vi "Mode_select_global_BM.vi"() -> ()   [LabVIEW 2021]
panel:
  in  "Mode Selection":T1(ring)
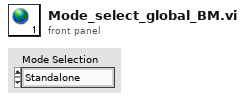
[diagram p1: front panel]
types:
  T1 = enum16{"Standalone", "Analysis", "Standard Curve", "Point Std"}
diagram:
